vi "DAQ.Create DAQmx Async Write.vi"(8 "error in (no error)":errorcluster, 11 "Array":refnum<k21>[](array[refnum])) -> (0 "error out":errorcluster, 3 "VI out":refnum<vi>)   [LabVIEW 2019, in "DAQmx.lvclass"]
uses:
  DAQmx.lvclass
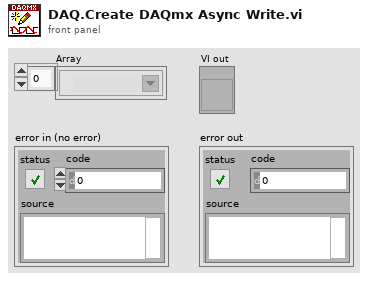
[diagram p1: front panel]
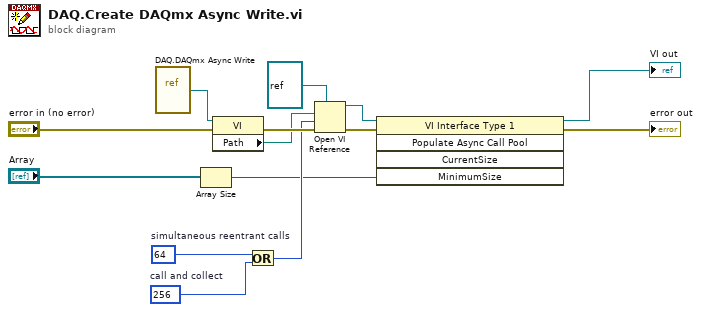
[diagram p0: block diagram]
diagram:
  w4 = 64  # simultaneous reentrant calls
  w3 = 256  # call and collect
  n1 = vi-ref "DAQ.DAQmx Async Write.vi"() -> (w1:refnum<vi>)
  n2 = Array Size(array="Array") -> (size(s)=w2:i32)
  n3 = property class="VI"(reference=w1, error in="error in (no error)") -> (error out=w7:errorcluster, "Path"=w6:path)  [unwired: 1 out]
  n4 = Or(x=w4, y=w3) -> (x .or. y?=w5:i32)
  n5 = Open VI Reference(type specifier VI Refnum (for type only)=refnum<vi> refnum, vi path=w6, options=w5, error in (no error)=w7) -> (vi reference=w9:refnum<vi>, error out=w10:errorcluster)  [unwired: 2 in]
  n6 = invoke class="VI Interface Type 1" method="Populate Async Call Pool"(reference=w9, error in=w10, "MinimumSize"=w2) -> (reference out=→"VI out":refnum<vi>, error out=→"error out":errorcluster)  [unwired: 2 in, 3 out]
